vi "Waveforms Generation GUID Lookup.vi"() -> ()   [LabVIEW 2013, in "Waveforms Generation Custom Device.lvlib"]
doc: "Use this Global VI to access the GUIDs assigned to the page resources of the Custom Device."
uses:
  Waveforms Generation Custom Device.lvlib
panel:
  in  "Waveform Page":string="14dba85d-898f-45ce-b8bb-981bf39eb0db"
  in  "Status Channel Page":string="8bd3ed4f-f3a1-4ee8-a28d-8c1c01f6f3b8"
  in  "Status Section Page":string="c49ecf0c-0d46-456e-844b-aa84eff493c3"
  in  "Waveform Property Channel Page":string="6c390138-a2b0-431d-b25e-04e5d2aad3b3"
  in  "Waveform Section Page":string="719c3d3c-fcb1-4ac0-9117-fc2552f9bccd"
  in  "Custom Device":string="9f4e723e-5d9b-47f0-9f55-5f71358bda74"
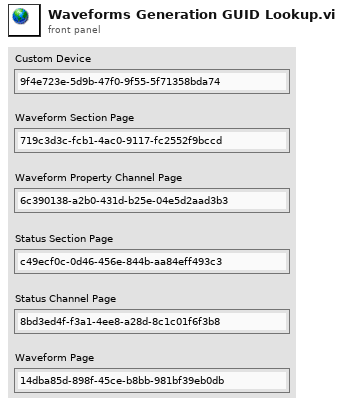
[diagram p1: front panel]
diagram:
